vi "Calculate conductance ITX.vi"(3 "single ended?":bool=TRUE, 4 "progress bar?":bool, 5 "length":i32=1, 7 "offset":i32, 9 "index":T2={"N1"=11, "N2"=19, "N3"=4, "N4"=5, "V1"=6, "V2"=4, "V3"=10, "V4"=13, "CURRENT"=7, "Vsg"=3}, 10 "File or Folder Path":path=path "P:/users1/kirkendall/data/SA02703M.20141112/7 - sweep Vsg, B") -> (0 "N Array":T1(array[cluster])=[{"N1"=0.0004, "N2"=0.0, "N3"=-6.47341032097701e-05, "N4"=-0.010645337299978234}], 1 "Comments":string="IGOR\nX// Date: 11/14/2014 5:01 PM\nX// SA02703M.20141112\nX// \nX// differential \nX// \nX// Vbg=-2.36V\nX// sweep Vsg: -100mV to 200mV, 1mV steps\nX// sweep B: sweep B 16T to -16T, 0.5T steps\nX// \nX// lockin\nX// 0: 3\nX// 1: 4, bad\nX// 2: 5\nX// 3: 7, curent \nX// 4: 9,\nX// 5: 2, current 5mV AC -190uV DC 400mHz\nX// appliedField= 16.000000\nX// appliedVsg= -0.100000\n\n\n\n\n\n\n\n\n\n\n\n\n\n\n\n\n\n\n\n\n\n\n\n\n\n\n\n\n\n\n\n\n\n\n\n\n\n\n\n\nX \nX Display/R 'time.SA02703M.20141112.0000'\nX AppendToGraph 'temp.SA02703M.20141112.0000'\nX AppendToGraph 'B.SA02703M.20141112.0000'\nX AppendToGraph 'Vsource.SA02703M.20141112.0000'\nX AppendToGraph 'Lockin0.SA02703M.20141112.0000'\nX AppendToGraph 'Lockin1.SA02703M.20141112.0000'\nX AppendToGraph 'Lockin2.SA02703M.20141112.0000'\nX AppendToGraph 'Lockin3.SA02703M.20141112.0000'\nX AppendToGraph 'Lockin4.SA02703M.20141112.0000'\nX AppendToGraph 'Lockin5.SA02703M.20141112.0000'\nX AppendToGraph 'B_rate.SA02703M.20141112.0000'\nX AppendToGraph 'DC0.SA02703M.20141112.0000'\nX AppendToGraph 'DC1.SA02703M.20141112.0000'\nX AppendToGraph 'DC2.SA02703M.20141112.0000'\nX AppendToGraph 'DC3.SA02703M.20141112.0000'\nX AppendToGraph 'DC4.SA02703M.20141112.0000'\nX AppendToGraph 'DC5.SA02703M.20141112.0000'\nX AppendToGraph 'DC6.SA02703M.20141112.0000'\nX AppendToGraph 'DC7.SA02703M.20141112.0000'\nX Label bottom \"x label\"\nX Label left \"y label\"\nX ModifyGraph rgb('time.SA02703M.20141112.0000')=(65280,0,0)\nX ModifyGraph rgb('temp.SA02703M.20141112.0000')=(65280,18432,0)\nX ModifyGraph rgb('B.SA02703M.20141112.0000')=(65280,36864,0)\nX ModifyGraph rgb('Vsource.SA02703M.20141112.0000')=(65280,55296,0)\nX ModifyGraph rgb('Lockin0.SA02703M.20141112.0000')=(57344,65280,0)\nX ModifyGraph rgb('Lockin1.SA02703M.20141112.0000')=(37376,65280,0)\nX ModifyGraph rgb('Lockin2.SA02703M.20141112.0000')=(18944,65280,0)\nX ModifyGraph rgb('Lockin3.SA02703M.20141112.0000')=(512,65280,0)\nX ModifyGraph rgb('Lockin4.SA02703M.20141112.0000')=(0,65280,17920)\nX ModifyGraph rgb('Lockin5.SA02703M.20141112.0000')=(0,65280,36352)\nX ModifyGraph rgb('B_rate.SA02703M.20141112.0000')=(0,65280,54784)\nX ModifyGraph rgb('DC0.SA02703M.20141112.0000')=(0,57856,65280)\nX ModifyGraph rgb('DC1.SA02703M.20141112.0000')=(0,39424,65280)\nX ModifyGraph rgb('DC2.SA02703M.20141112.0000')=(0,20992,65280)\nX ModifyGraph rgb('DC3.SA02703M.20141112.0000')=(0,2560,65280)\nX ModifyGraph rgb('DC4.SA02703M.20141112.0000')=(17408,0,65280)\nX ModifyGraph rgb('DC5.SA02703M.20141112.0000')=(35840,0,65280)\nX ModifyGraph rgb('DC6.SA02703M.20141112.0000')=(54272,0,65280)\nX ModifyGraph rgb('DC7.SA02703M.20141112.0000')=(65280,0,58368)\nX Legend/C/N=text0/J \"\\\\s('time.SA02703M.20141112.0000') time\\r\\\\s('temp.SA02703M.20141112.0000') temp\\r\\\\s('B.SA02703M.20141112.0000') B\\r\\\\s('Vsource.SA02703M.20141112.0000') Vsource\\r\\\\s('Lockin0.SA02703M.20141112.0000') Lockin0\\r\\\\s('Lockin1.SA02703M.20141112.0000') Lockin1\\r\\\\s('Lockin2.SA02703M.20141112.0000') Lockin2\\r\\\\s('Lockin3.SA02703M.20141112.0000') Lockin3\\r\\\\s('Lockin4.SA02703M.20141112.0000') Lockin4\\r\\\\s('Lockin5.SA02703M.20141112.0000') Lockin5\\r\\\\s('B_rate.SA02703M.20141112.0000') B_rate\\r\\\\s('DC0.SA02703M.20141112.0000') DC0\\r\\\\s('DC1.SA02703M.20141112.0000') DC1\\r\\\\s('DC2.SA02703M.20141112.0000') DC2\\r\\\\s('DC3.SA02703M.20141112.0000') DC3\\r\\\\s('DC4.SA02703M.20141112.0000') DC4\\r\\\\s('DC5.SA02703M.20141112.0000') DC5\\r\\\\s('DC6.SA02703M.20141112.0000') DC6\\r\\\\s('DC7.SA02703M.20141112.0000') DC7\"\nX ModifyGraph mirror(bottom)=1\nX ModifyGraph width=216\nX ModifyGraph height={Aspect,0.6}\nX ModifyGraph Log(bottom)=0\nX ModifyGraph Log(left)=0\nX \n", 2 "A vs D diff":cluster{dbl[], dbl[]}[](graph), 6 "angle phi":dbl[](array[numeric])=[179.65158969757934], 8 "angle theta":dbl[](array[numeric])=[-90.0], 11 "A vs D":cluster{dbl[], dbl[]}[](graph))   [LabVIEW 2020, in "Tranconductance SM.lvclass"]
uses:
  Tranconductance SM.lvclass
  <vilib>/Analysis/NI_AALPro.lvlib
  <vilib>/addons/WireFlow/_WF_ProgressBar.llb/ProgressBar_WireFlow.lvclass
  <userlib>/LevyLab/Graph Utilities/graph_utilities.lvclass
  <userlib>/LevyLab/LV-Data/LV-Data/LV-Data.lvclass
  <userlib>/LevyLab/XY Utilities/xy_utilities.lvlib
  <userlib>/LevyLab/XY Utilities/subVIs/Derivative (single).vi
  <vilib>/Utility/miscctls.llb/LVOffsetAndMultiplierTypeDef.ctl
panel:
  out "WF-ProgressBar out":refnum<class "ProgressBar_WireFlow.lvclass">
  in  "Enum":enum16{"Conductance", "Resistance", "Current"}(ring)
  in  "alpha":dbl=0.00528086 format="%#_13g"
  in  "alpha?":bool
  in  "Numeric":dbl=50.0
  in  "Type":enum16{"dy/dx vs x", "dx/dy vs y"}(ring)
  in  "e^2/h?":bool=TRUE
  in  "log scale?":bool
  in  "calculate Ey":bool=TRUE
  in  "background":enum16{"do nothing", "subtract", "divide"}(ring)
  in  "Background":cluster{dbl[], dbl[]}[](graph)
  in  "A offset":dbl format="%#_6p"
  out "E 2":dbl[][](graph)
  out "counter":i32
  out "Path":path=path "P:/users1/kirkendall/data/SA02703M.20141112/7 - sweep Vsg, B/SA02703M.20141112.0000.itx"
  out "Index, Wavenames":string[][](table)=[["0", "'time.SA02703M.20141112.0000'\n"], ["1", "'temp.SA02703M.20141112.0000'\n"], ["2", "'B.SA02703M.20141112.0000'\n"], ["3", "'Vsource.SA02703M.20141112.0000'\n"], ["4", "'Lockin0.SA02703M.20141112.0000'\n"], ["5", "'Lockin1.SA02703M.20141112.0000'\n"], ["6", "'Lockin2.SA02703M.20141112.0000'\n"], ["7", "'Lockin3.SA02703M.20141112.0000'\n"], ["8", "'Lockin4.SA02703M.20141112.0000'\n"], ["9", "'Lockin5.SA02703M.20141112.0000'\n"], ["10", "'B_rate.SA02703M.20141112.0000'\n"], ["11", "'DC0.SA02703M.20141112.0000'\n"], ["12", "'DC1.SA02703M.20141112.0000'\n"], ["13", "'DC2.SA02703M.20141112.0000'\n"], ["14", "'DC3.SA02703M.20141112.0000'\n"], ["15", "'DC4.SA02703M.20141112.0000'\n"], ["16", "'DC5.SA02703M.20141112.0000'\n"], ["17", "'DC6.SA02703M.20141112.0000'\n"], ["18", "'DC7.SA02703M.20141112.0000'\n"], ["", ""]]
  out "N":cluster{"N1":dbl, "N2":dbl, "N3":dbl, "N4":dbl}={"N1"=0.0004, "N2"=0.0, "N3"=-6.47341032097701e-05, "N4"=-0.010645337299978234} {"N4" format="%#_6p"; "N3" format="%#_6p"; "N2" format="%#_6p"; "N1" format="%#_20p"}
  in  "Ey":T3={"Offset"=0.0, "Multiplier"=1.0}
  in  "Ex":T3={"Offset"=0.0, "Multiplier"=1.0}
  out "C vs D":cluster{dbl[], dbl[]}[](graph)
  out "E":dbl[][](graph)
  in  "B x name":string="Vsg (V)"
  in  "A y name":string="Conductance (S)"
  in  "Ex name":string="Ex name"
  in  "Ez name":string="Ez name"
  in  "D x name":string="Vsg (V)"
  in  "C y name":string="Conductance (S)"
  in  "Ey name":string="Ey name"
  out "time":string[][](table)=[["11/14/2014", "5:01 PM"]]
  in  "B is time?":bool
  in  "D  is time?":bool
  in  "pattern":string="*.itx"
  # "CURRENT/(V1-V2)"
  # "CURRENT/(V3-V4)"
  # "x axis: Vsg\ny axis: single ended?\nT: subtract V1-V2 and V3-V4 and divide by current\nF: plot V1/current"
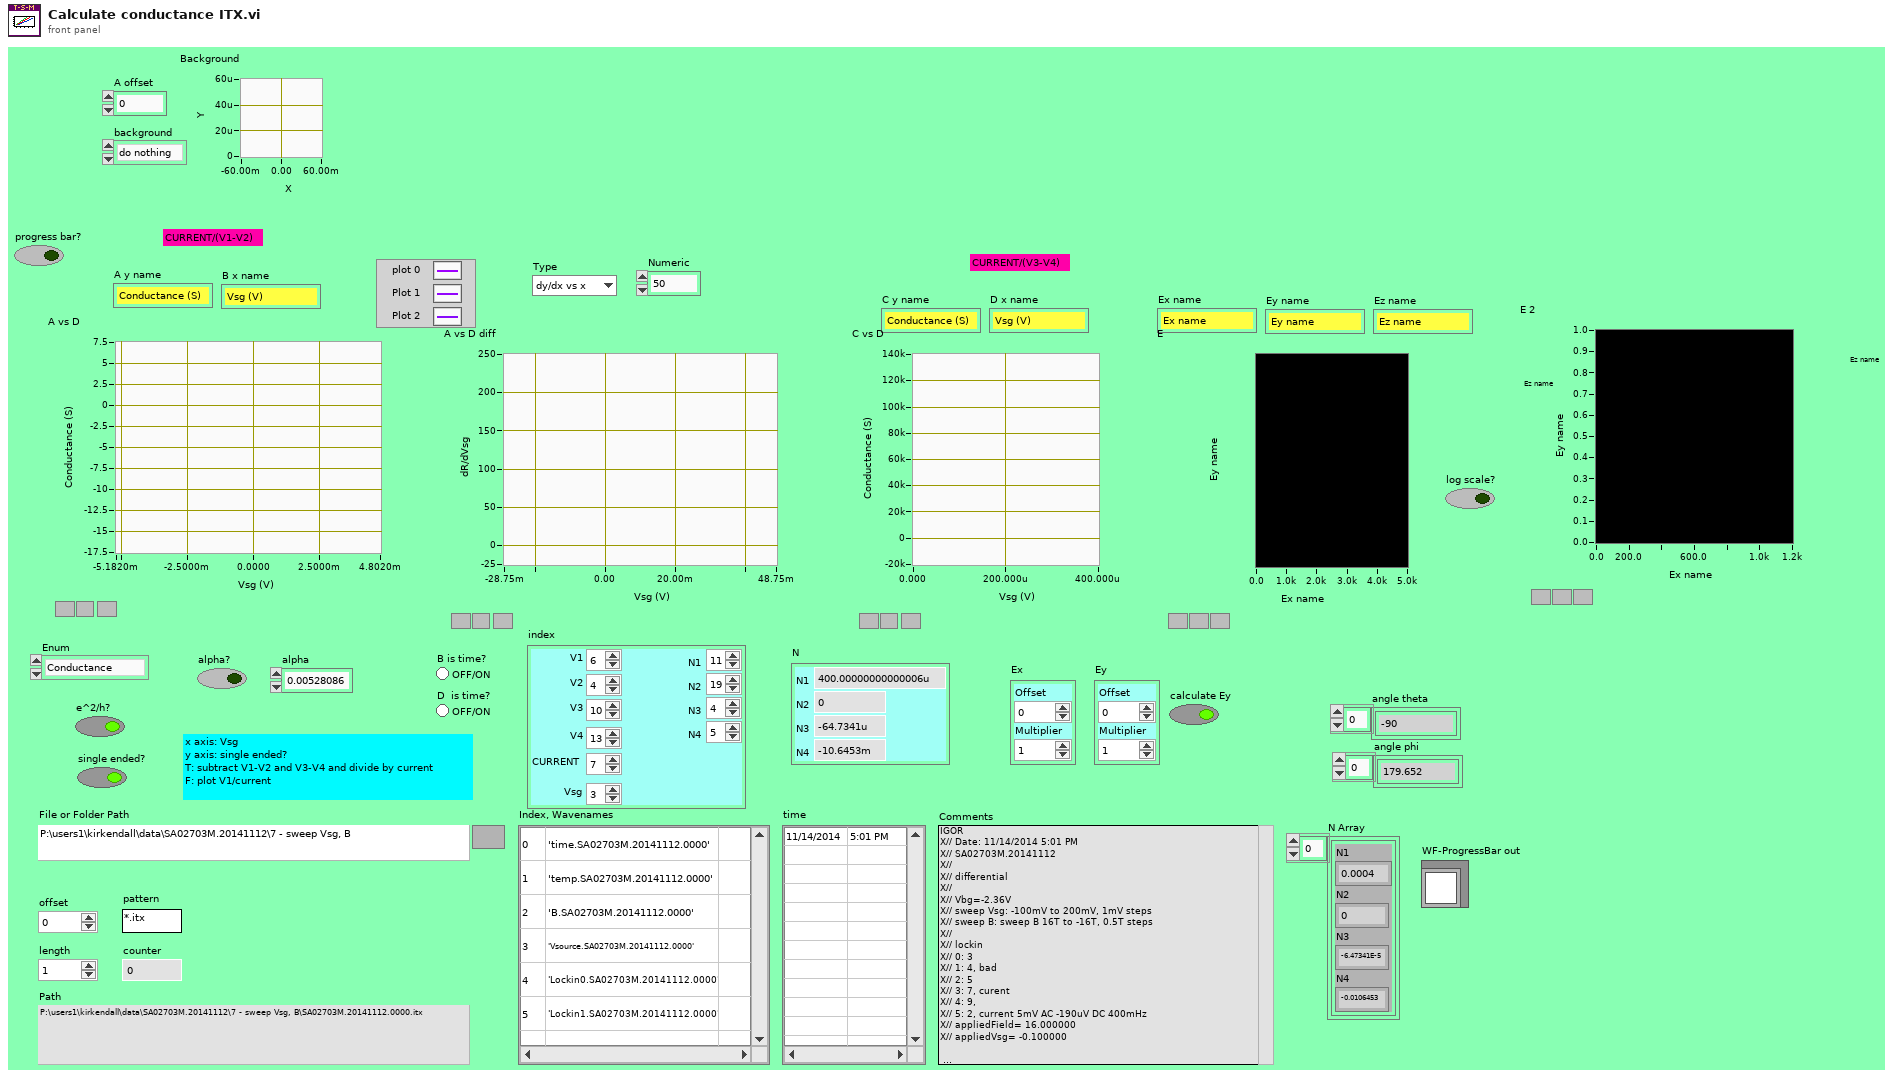
[diagram p1: front panel]
types:
  T1 = cluster{"N1":dbl, "N2":dbl, "N3":dbl, "N4":dbl}[]
  T2 = cluster{"N1":i32, "N2":i32, "N3":i32, "N4":i32, "V1":i32, "V2":i32, "V3":i32, "V4":i32, "CURRENT":i32, "Vsg":i32}
  T3 = typedef "LVOffsetAndMultiplierTypeDef.ctl" = cluster{"Offset":dbl, "Multiplier":dbl}
  T4 = typedef "LV-Data.lvclass/Dictionary--cluster.ctl" = cluster{"key":string, "value":variant}
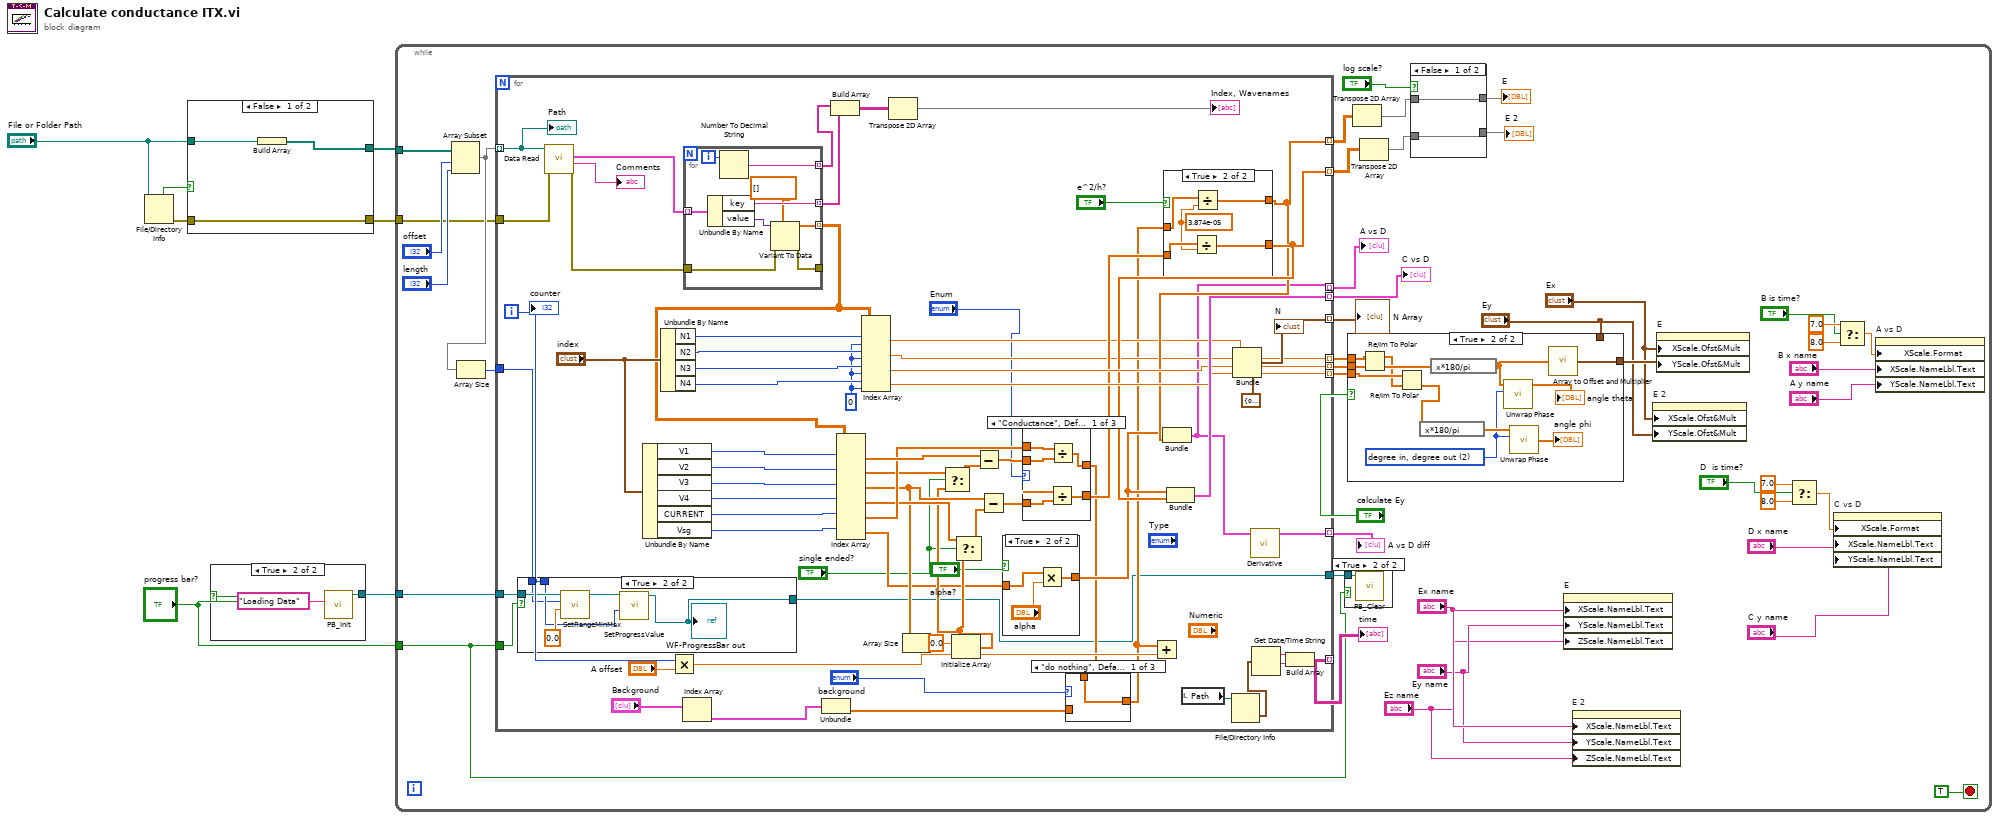
[diagram p0: block diagram]
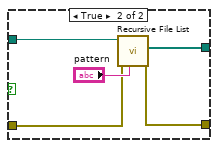
[diagram p2: hidden frame]
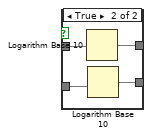
[diagram p5: hidden frame]
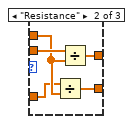
[diagram p10: hidden frame]
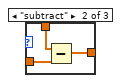
[diagram p12: hidden frame]
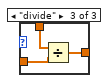
[diagram p13: hidden frame]
diagram:
  n1 = File/Directory Info(path="File or Folder Path") -> (directory=w2:bool, error out=w1:errorcluster)  [unwired: 1 in, 5 out]
  n2 = case shown="False" w2 {
    tunnel: [w10 w14] -> w6
    tunnel: "File or Folder Path" -> [w9 w13]
    tunnel: [w8 w11] -> w3
    tunnel: w1 -> [w8 w12]
    frame False {
      n3 = Build Array(w9) -> (w10:path[])
    }
    frame True {
      n4 = call <vilib>:"Recursive File List.vi"("pattern"="pattern", "error in (no error)"=w12, "Folder Path"=w13) -> ("error out"=w11:errorcluster, "All Files in Dir"=w14:path[])  [unwired: 4 in, 3 out]
    }
  }
  n5 = case shown="True" "progress bar?" {
    tunnel: [_ w17] -> w5
    frame False {
    }
    frame True {
      n6 = call <vilib>:"PB_Init.vi"("title (\"Progress\")"="Loading Data" ("title (\"Progress\")")) -> ("WF-ProgressBar out"=w17:refnum<class "ProgressBar_WireFlow.lvclass">)  [unwired: 9 in, 1 out]
    }
  }
  n7 = while {
    tunnel: w6 -> [w55]
    tunnel: w5 -> [w26]
    tunnel: "progress bar?" -> [w21]
    tunnel: w3 -> [w20]
    stop <- TRUE stop-if-true
    n8 = Array Subset(array=w55, index="offset", length="length") -> (w24:path[])
    n9 = Array Size(array=w24) -> (size(s)=w23:i32)
    n10 = for {
      tunnel: w24 -> [w151] mode=indexing
      tunnel: [w151] -> _ mode=indexing
      tunnel: [w139] -> w57 mode=indexing
      tunnel: [w83] -> w46 mode=indexing
      tunnel: [w127] -> w47 mode=indexing
      tunnel: [w114] -> w45 mode=indexing
      tunnel: [w115] -> w44 mode=indexing
      tunnel: [w103] -> w39 mode=indexing
      tunnel: [w119] -> w38 mode=indexing
      tunnel: [w118] -> w37 mode=indexing
      tunnel: [w113] -> w28 mode=indexing
      tunnel: [w82] -> w27 mode=indexing
      tunnel: w26 -> [w95]
      tunnel: w23 -> [w93]
      tunnel: [w92] -> w22
      tunnel: w21 -> [w91]
      tunnel: w20 -> [w88]
      i -> [w94]
      w137 = 0 ("disabled index (col)")
      n11 = case shown="True" w91 {
        tunnel: w95 -> [_ w166]
        tunnel: w94 -> [_ w163]
        tunnel: w93 -> [_ w162]
        tunnel: [_ w161] -> w92
        frame False {
        }
        frame True {
          n12 = call-dynamic "SetRangeMinMax.vi"("Min (0)"=0.0, "Max (1)"=w162, "WF-ProgressBar in"=w166) -> ("WF-ProgressBar out"=w164:refnum<class "ProgressBar_WireFlow.lvclass">)  [unwired: 7 in, 1 out]
          n13 = call-dynamic "SetProgressValue.vi"("Value"=w163, "WF-ProgressBar in"=w164) -> ("WF-ProgressBar out"=w161:refnum<class "ProgressBar_WireFlow.lvclass">)  [unwired: 7 in, 2 out]
          "WF-ProgressBar out" <- w161
        }
      }
      n14 = call <userlib>:"Data Read.vi"("error in (no error)"=w88, "path"=w151) -> ("error out"=w87:errorcluster, "Notes"=→"Comments":string, "Data (Dictionary)"=w90:T4[])  [unwired: 6 in, 1 out]
      n15 = Unbundle By Name("index") -> ("V1"=w136:i32, "V2"=w135:i32, "V3"=w134:i32, "V4"=w133:i32, "CURRENT"=w131:i32, "Vsg"=w126:i32)
      n16 = Unbundle By Name("index") -> ("N1"=w144:i32, "N2"=w145:i32, "N3"=w146:i32, "N4"=w147:i32)
      n17 = Multiply(x=w94, y="A offset") -> (x*y=w124:dbl)
      n18 = Index Array(array="Background") -> (element=w121:cluster{dbl[], dbl[]})  [unwired: 1 in]
      n19 = for {
        tunnel: [w159] -> w85 mode=indexing
        tunnel: w90 -> [w158] mode=indexing
        tunnel: [w157] -> w86 mode=indexing
        tunnel: [w155] -> w89 mode=indexing
        tunnel: w87 -> [w153]
        tunnel: [w152] -> _
        i -> [w160]
        n20 = Unbundle By Name(w158) -> ("key"=w157:string, "value"=w154:variant)
        n21 = Number To Decimal String(number=w160) -> (decimal integer string=w159:string)  [unwired: 1 in]
        n22 = Variant To Data(error in=w153, type=dbl[] [], Variant=w154) -> (data=w155:dbl[], error out=w152:errorcluster)
      }
      n23 = Unbundle(w121) -> (w122:dbl[])  [unwired: 1 out]
      n24 = Build Array(w85, w86) -> (w149:string[][])
      n25 = Index Array(array=w89, index (row) #1=w136, index (row) #2=w135, index (row) #3=w134, index (row) #4=w133, index (row) #5=w131, index (row) #6=w126) -> (element #1=w132:dbl[], element #2=w112:dbl[], element #3=w108:dbl[], element #4=w110:dbl[], element #5=w129:dbl[], element #6=w101:dbl[])  [unwired: 6 in]
      n26 = Index Array(array=w89, index (row) #1=w144, index (col) #1=w137, index (row) #2=w145, index (col) #2=w137, index (row) #3=w146, index (col) #3=w137, index (row) #4=w147, index (col) #4=w137) -> (element #1=w104:dbl, element #2=w103:dbl, element #3=w119:dbl, element #4=w118:dbl)
      n27 = Transpose 2D Array(2D array=w149) -> (transposed array=→"Index, Wavenames":string[][])
      n28 = Array Size(array=w108) -> (size(s)=w106:i32)
      n29 = Initialize Array(0.0 ("element"), w106) -> (w105:dbl[])
      n30 = Select(t=w112, s="single ended?", f=w105) -> (s? t:f=w111:dbl[])
      n31 = Select(t=w110, s="single ended?", f=w105) -> (s? t:f=w109:dbl[])
      n32 = Subtract(x=w132, y=w111) -> (x-y=w130:dbl[])
      n33 = Subtract(x=w108, y=w109) -> (x-y=w128:dbl[])
      n34 = case shown="True" "alpha?" {
        tunnel: w101 -> [w167 w170]
        tunnel: [w167 w169] -> w100
        frame False {
        }
        frame True {
          n35 = Multiply(x=w170, y="alpha") -> (x*y=w169:dbl[])
        }
      }
      n36 = case shown="\"Conductance\", Default" "Enum" {
        tunnel: w130 -> [w182 w187 _]
        tunnel: w129 -> [w181 w185 w188]
        tunnel: w128 -> [w180 w184 _]
        tunnel: [w179 w183 w188] -> w117
        tunnel: [w178 w186 w188] -> w98
        frame "Conductance", Default {
          n37 = Divide(x=w181, y=w180) -> (x/y=w179:dbl[])
          n38 = Divide(x=w181, y=w182) -> (x/y=w178:dbl[])
        }
        frame "Resistance" {
          n39 = Divide(x=w184, y=w185) -> (x/y=w183:dbl[])
          n40 = Divide(x=w187, y=w185) -> (x/y=w186:dbl[])
        }
        frame "Current" {
        }
      }
      n41 = case shown="\"do nothing\", Default" "background" {
        tunnel: w98 -> [w189 w192 w195]
        tunnel: [w189 w191 w193] -> w99
        tunnel: w122 -> [_ w190 w194]
        frame "do nothing", Default {
        }
        frame "subtract" {
          n42 = Subtract(x=w192, y=w190) -> (x-y=w191:dbl[])
        }
        frame "divide" {
          n43 = Divide(x=w195, y=w194) -> (x/y=w193:dbl[])
        }
      }
      n44 = Add(x=w99, y=w124) -> ()  [unwired: 1 out]
      n45 = case shown="True" "e^2/h?" {
        tunnel: w117 -> [w171 w175]
        tunnel: w99 -> [w172 w177]
        tunnel: [w172 w176] -> w114
        tunnel: [w171 w174] -> w115
        frame False {
        }
        frame True {
          w173 = 3.874e-05
          n46 = Divide(x=w175, y=w173) -> (x/y=w174:dbl[])
          n47 = Divide(x=w177, y=w173) -> (x/y=w176:dbl[])
        }
      }
      n48 = Bundle(w100, w114) -> (w83:cluster{dbl[], dbl[]})  [unwired: 1 in]
      n49 = Bundle(w100, w115) -> (w127:cluster{dbl[], dbl[]})  [unwired: 1 in]
      n50 = local read "Path"() -> (w143:path)
      n51 = File/Directory Info(path=w143) -> (last mod=w142:timestamp)  [unwired: 1 in, 6 out]
      n52 = Bundle(cluster=cluster{"N1":dbl, "N2":dbl, "N3":dbl, "N4":dbl} {"N1"=0.0, "N2"=0.0, "N3"=0.0, "N4"=0.0}, "N1"=w104, "N2"=w103, "N3"=w119, "N4"=w118) -> (w113:cluster{"N1":dbl, "N2":dbl, "N3":dbl, "N4":dbl})
      "N" <- w113
      n53 = call-poly <userlib>:"Derivative.vi"("XY-data"=w83) -> ("XY-data out"=w82:cluster{"X-array":dbl[], "Y-array":dbl[]})  [unwired: 8 in, 2 out]
      n54 = Get Date/Time String(seconds (now)=w142) -> (date string=w141:string, time string=w140:string)  [unwired: 2 in]
      n55 = Build Array(w141, w140) -> (w139:string[])
      "counter" <- w94
      "Path" <- w151
    }
    "A vs D" <- w46
    "C vs D" <- w47
    "time" <- w57
    "N Array" <- w28
    "A vs D diff" <- w27
    n56 = case shown="True" w21 {
      tunnel: w22 -> [_ w62]
      frame False {
      }
      frame True {
        n57 = call-dynamic "PB_Clear.vi"("WF-ProgressBar in"=w62) -> ()  [unwired: 9 in, 2 out]
      }
    }
    n58 = case shown="True" "calculate Ey" {
      tunnel: w39 -> [_ w81]
      tunnel: w38 -> [_ w80]
      tunnel: w37 -> [_ w75]
      tunnel: [w69 w73] -> w36
      tunnel: "Ey" -> [w69 _]
      frame False {
      }
      frame True {
        w71 = 2 items=["radian in, radian out", "radian in, degree out", "degree in, degree out", "degree in, radian out"] ("phase unit")
        n59 = Re/Im To Polar(2:w80, 3:w81) -> (0:w79:dbl[], 1:w74:dbl[])
        n60 = Re/Im To Polar(2:w74, 3:w75) -> (0:w70:dbl[])  [unwired: 1 out]
        n61 = expression code="x*180/pi"(w70) -> (w77:dbl[])
        n62 = expression code="x*180/pi"(w79) -> (w72:dbl[])
        n63 = call <vilib>:"Unwrap Phase.vi"("phase unit"=w71, "Phase"=w72) -> ("Unwrapped Phase"=→"angle theta":dbl[])  [unwired: 8 in, 1 out]
        n64 = call <vilib>:"Unwrap Phase.vi"("phase unit"=w71, "Phase"=w77) -> ("Unwrapped Phase"=→"angle phi":dbl[])  [unwired: 8 in, 1 out]
        n65 = call <userlib>:"Array to Offset and Multiplier.vi"("Array"=w72) -> ("Offset and Multiplier"=w73:T3)
      }
    }
    n66 = Transpose 2D Array(2D array=w45) -> (transposed array=w32:dbl[][])
    n67 = Transpose 2D Array(2D array=w44) -> (transposed array=w30:dbl[][])
    n68 = case shown="False" "log scale?" {
      tunnel: w32 -> [w64 w68]
      tunnel: [w64 w67] -> w31
      tunnel: w30 -> [w63 w66]
      tunnel: [w63 w65] -> w29
      frame False {
      }
      frame True {
        n69 = Logarithm Base 10(1:w68) -> (0:w67:dbl[][])
        n70 = Logarithm Base 10(1:w66) -> (0:w65:dbl[][])
      }
    }
    "E" <- w31
    "E 2" <- w29
    n71 = property on="E" class="IntGraph (strict)"("XScale.NameLbl.Text"="Ex name", "YScale.NameLbl.Text"="Ey name", "ZScale.NameLbl.Text"="Ez name") -> ()  [unwired: 2 in, 2 out]
    n72 = property on="E 2" class="IntGraph (strict)"("XScale.NameLbl.Text"="Ex name", "YScale.NameLbl.Text"="Ey name", "ZScale.NameLbl.Text"="Ez name") -> ()  [unwired: 2 in, 2 out]
    n73 = property on="E 2" class="IntGraph (strict)"("XScale.Ofst&Mult"="Ex", "YScale.Ofst&Mult"="Ey") -> ()  [unwired: 2 in, 2 out]
    n74 = property on="E" class="IntGraph (strict)"("XScale.Ofst&Mult"="Ex", "YScale.Ofst&Mult"=w36) -> ()  [unwired: 2 in, 2 out]
    n75 = Select(t=7.0, s="D  is time?", f=8.0) -> (s? t:f=w51:dbl)
    n76 = property on="C vs D" class="XYGraph (strict)"("XScale.Format"=w51, "XScale.NameLbl.Text"="D x name", "YScale.NameLbl.Text"="C y name") -> ()  [unwired: 2 in, 2 out]
    n77 = Select(t=7.0, s="B is time?", f=8.0) -> (s? t:f=w52:dbl)
    n78 = property on="A vs D" class="XYGraph (strict)"("XScale.Format"=w52, "XScale.NameLbl.Text"="B x name", "YScale.NameLbl.Text"="A y name") -> ()  [unwired: 2 in, 2 out]
  }
